vi "Update.vi"(8 "error in (no error)":errorcluster, 10 "Message in":refnum<class "UpdateMessage.lvclass">, 11 "LineCCD in":refnum<class "LineCCD.lvclass">) -> (0 "error out":errorcluster, 3 "LineCCD out":refnum<class "LineCCD.lvclass">)   [LabVIEW 2012, in "LineCCD.lvclass"]
doc: "The update method processes the command 'update'. \n\nThe command 'update' is used for receiving new values to be set to the private data of the class. This could be seen as a public set method for setting new parameters to the private class data."
uses:
  LineCCD.lvclass
  <vilib>/Distrio/Murmex/Murmex/Murmex.lvclass
  <vilib>/Distrio/Murmex/UpdateMessage/UpdateMessage.lvclass
panel:
  # "This method is called when the UPDATE\ntrigger is sent. \n\nOverride this method when your component needs to\nrespond to this trigger. \n\nCall parent for proper implementation"
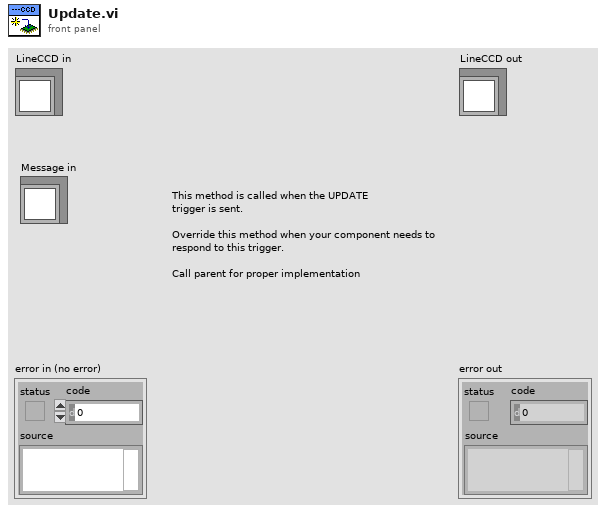
[diagram p1: front panel]
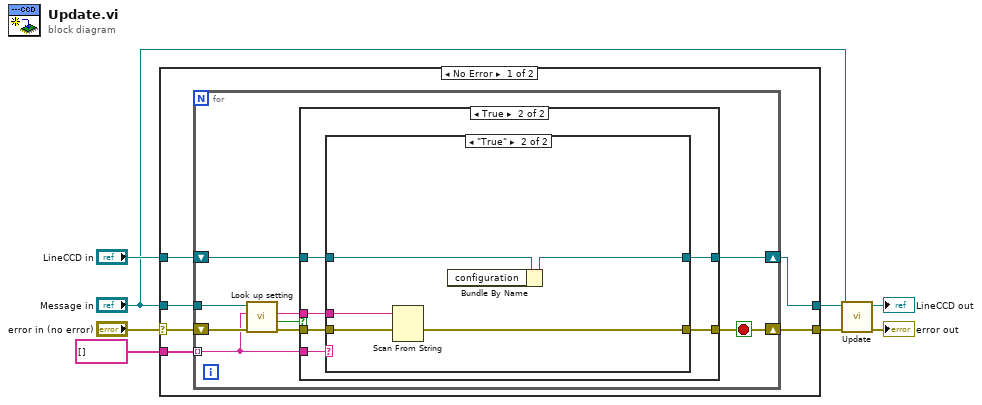
[diagram p0: block diagram]
diagram:
  n1 = case shown="No Error" "error in (no error)" {
    selector: "error in (no error)" -> [w14 w39]
    tunnel: "LineCCD in" -> [w13 w40]
    tunnel: "Message in" -> [w12 _]
    tunnel: string[] [] -> [w11 _]
    tunnel: [w10 w39] -> w2
    tunnel: [w9 w40] -> w1
    frame No Error {
      n2 = for {
        shift-right: [w15] -> w10
        shift-left: w14 -> [w23]
        shift-right: [w16] -> w9
        shift-left: w13 -> [w17]
        tunnel: w12 -> [w22]
        tunnel: w11 -> [w18] mode=indexing
        stop <- w15 stop-if-true
        n3 = call <vilib>:"Look up setting.vi"("error in (no error)"=w23, "tag name"=w18, "UpdateMessage in"=w22) -> ("error out"=w21:errorcluster, "found?"=w20:bool, "value"=w19:string)  [unwired: 5 in, 1 out]
        n4 = case shown="True" w20 {
          tunnel: w21 -> [w24 w31]
          tunnel: w19 -> [_ w30]
          tunnel: w18 -> [_ w29]
          tunnel: w17 -> [w25 w28]
          tunnel: [w25 w26] -> w16
          tunnel: [w24 w27] -> w15
          frame False {
          }
          frame True {
            n5 = case shown="\"True\"" w29 {
              tunnel: w31 -> [w32 w38]
              tunnel: w30 -> [_ w37]
              tunnel: w28 -> [w33 w35]
              tunnel: [w32 w36] -> w27
              tunnel: [w33 w34] -> w26
              frame "False", Default {
              }
              frame "True" {
                n6 = Scan From String(input string=w37, error in=w38) -> (error out=w36:errorcluster)  [unwired: 4 in, 2 out]
                n7 = Bundle By Name(cluster=w35) -> (w34:refnum<class "LineCCD.lvclass">)  [unwired: 1 in]
              }
            }
          }
        }
      }
    }
    frame Error {
    }
  }
  n8 = call-parent "Update.vi"("error in (no error)"=w2, "Message in"="Message in", "Murmex in"=w1) -> ("error out"=→"error out":errorcluster, "Murmex out"=→"LineCCD out":refnum<class "LineCCD.lvclass">)  [unwired: 7 in]
